vi "Actor Core.vi"(8 "error in":errorcluster, 11 "Sequencer in":refnum<class "Sequencer.lvclass">) -> (0 "error out":errorcluster, 3 "Actor out":refnum<class "Actor.lvclass">)   [LabVIEW 2015, in "Sequencer.lvlib" / "Sequencer.lvclass"]
doc: "(<B>Filename</B>: Actor Framework.lvlib:Actor.lvclass:Actor Core.vi)\n\nReceives messages to the actor, reacts to them, and initiates any error handling that may shut the actor down.\n\nDescendant classes may override this VI to append parallel tasks for the actor to complete while it handles messages. Overrides use the Call Parent Method node."
uses:
  Sequencer.lvclass
  <userlib>/_Win8uiFramework/ViewableActor.lvclass
  <vilib>/ActorFramework/Actor/Actor.lvclass
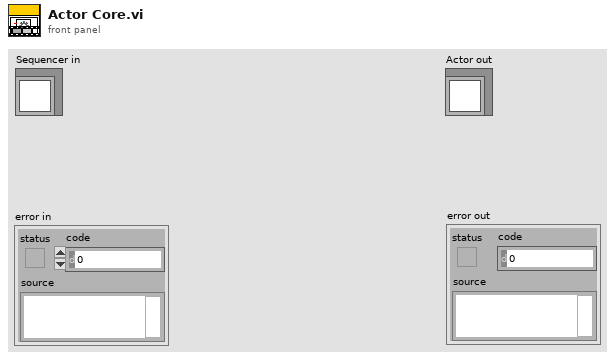
[diagram p1: front panel]
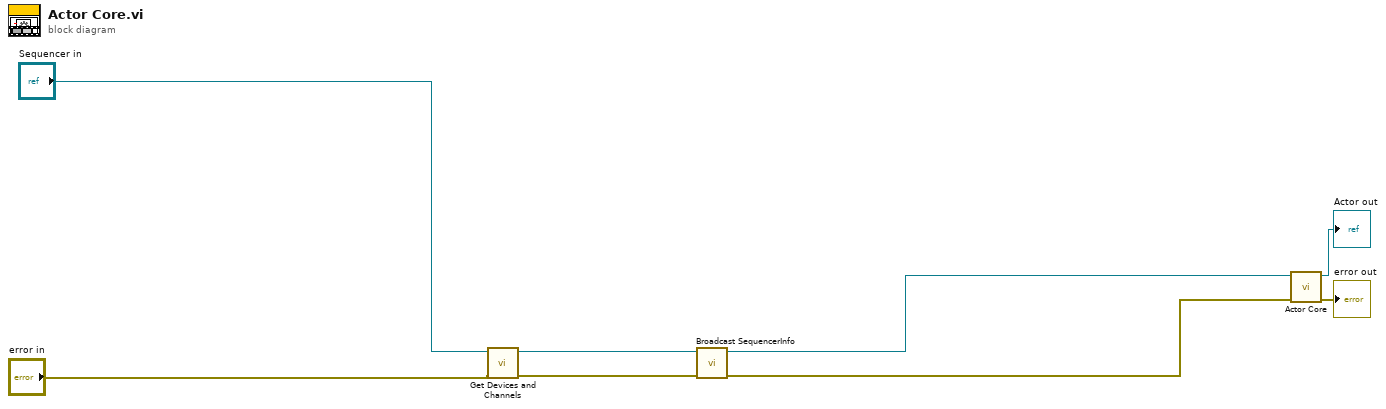
[diagram p0: block diagram]
diagram:
  n1 = call "Get Devices and Channels.vi"("error in (no error)"="error in", "Sequencer in"="Sequencer in") -> ("error out"=w4:errorcluster, "Sequencer out"=w2:refnum<class "Sequencer.lvclass">)  [unwired: 8 in]
  n2 = call "Broadcast SequencerInfo.vi"("error in (no error)"=w4, "Sequencer in"=w2) -> ("error out"=w3:errorcluster, "Sequencer out"=w1:refnum<class "Sequencer.lvclass">)  [unwired: 8 in]
  n3 = call-parent "Actor Core.vi"("error in"=w3, "Actor in"=w1) -> ("error out"=→"error out":errorcluster, "Actor out"=→"Actor out":refnum<class "Actor.lvclass">)  [unwired: 8 in]
